vi "Configure Instrument.vi"(8 "error in (no error)":errorcluster, 11 "Instrument.sample-registry":refnum<class "Instrument.sample-registry.lvclass">) -> (0 "error out":errorcluster, 3 "Instrument.sample-registry out":refnum<class "Instrument.sample-registry.lvclass">)   [LabVIEW 2019, in "Instrument.sample-registry.lvclass"]
uses:
  Instrument.sample-registry.lvclass
  <userlib>/LevyLab/Levylab Instruments/Instrument Types/VSource/Instrument.VSource.lvclass
panel:
  # "Use this if you want to \nhave a configuration\nwindow specific to your\ninstrument. Otherwise you\nmay delete"
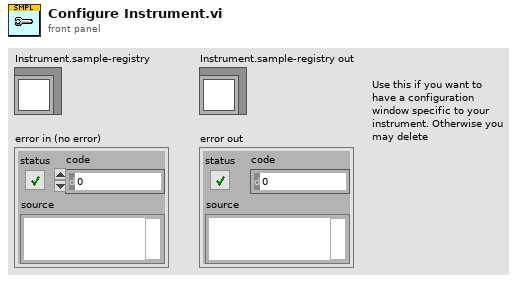
[diagram p1: front panel]
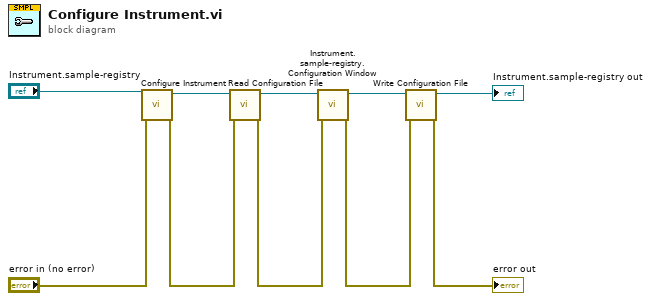
[diagram p0: block diagram]
diagram:
  n1 = call-parent "Configure Instrument.vi"("error in (no error)"="error in (no error)", "Instrument in"="Instrument.sample-registry") -> ("error out"=w5:errorcluster, "Instrument out"=w7:refnum<class "Instrument.sample-registry.lvclass">)  [unwired: 8 in]
  n2 = call-dynamic "Read Configuration File.vi"("error in (no error)"=w5, "Instrument.sample-registry"=w7) -> ("error out"=w4:errorcluster, "Instrument.sample-registry out"=w3:refnum<class "Instrument.sample-registry.lvclass">)  [unwired: 8 in]
  n3 = call "Instrument.sample-registry.Configuration Window.vi"("error in (no error)"=w4, "Instrument.sample-registry"=w3) -> ("error out"=w1:errorcluster, "Instrument.sample-registry out"=w2:refnum<class "Instrument.sample-registry.lvclass">)  [unwired: 8 in]
  n4 = call-dynamic "Write Configuration File.vi"("error in (no error)"=w1, "Instrument.sample-registry"=w2) -> ("error out"=→"error out":errorcluster, "Instrument.sample-registry out"=→"Instrument.sample-registry out":refnum<class "Instrument.sample-registry.lvclass">)  [unwired: 8 in]
